vi "Test Stop.vi"(11 "Error in":errorcluster) -> (15 "Error out":errorcluster)   [LabVIEW 2020, in "CelsiusToFarenheitTests.lvlib"]
doc: "This VI is to validate the stop button"
uses:
  CelsiusToFarenheitTests.lvlib
  <vilib>/addons/_JKI Toolkits/Caraya/classes/Test Suite/Define Test Suite (JUnit Report).vi
  <vilib>/SLL Drona/APIs/Assert/AssertVI/AssertVIExecRunning.vi
  <vilib>/SLL Drona/APIs/Stimulus/ControlValue/SetValueAuto.vi
  <vilib>/SLL Drona/APIs/Assert/AssertVI/AssertVIExecIdle.vi
  <vilib>/SLL Drona/APIs/Stimulus/VI/CloseVI.vi
  <vilib>/addons/_JKI Toolkits/Caraya/classes/Test Suite/Test Suite.lvclass
  <vilib>/SLL Drona/Drona.lvlib
  <vilib>/addons/_JKI Toolkits/Caraya/classes/Test/Test.lvclass
  <vilib>/SLL Drona/APIs/Assert/AssertVI/AssertVI.lvlib
  <vilib>/SLL Drona/APIs/Stimulus/ControlValue/ControlValue.lvlib
  <vilib>/SLL Drona/APIs/Stimulus/VI/VI.lvlib
  <vilib>/Wiresmith Technology/G CLI/CLI Class/CLI.lvclass
panel:
  # "STOP BUTTON TEST"
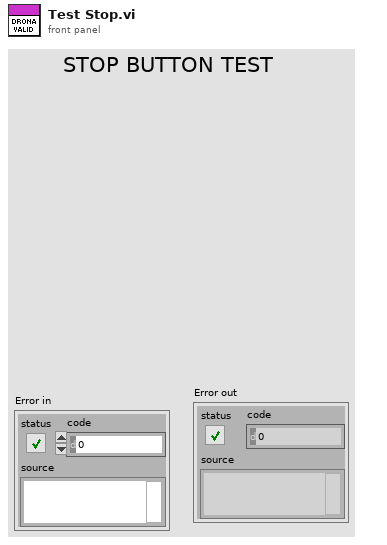
[diagram p1: front panel]
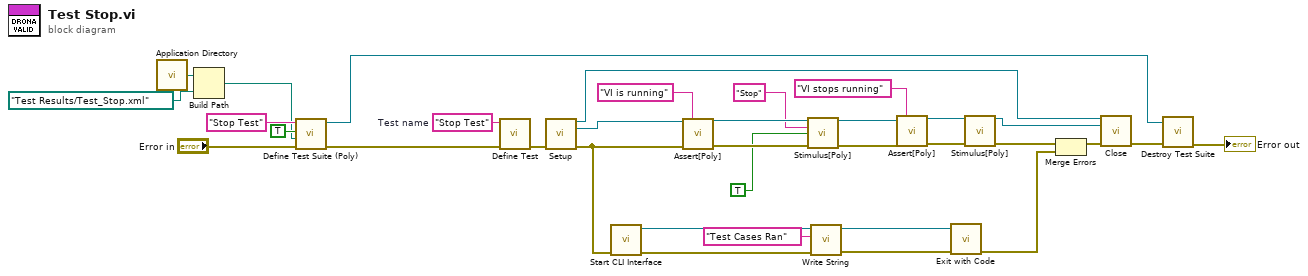
[diagram p0: block diagram]
diagram:
  w33 = "Stop Test"  # Test name
  n1 = call <vilib>:"Application Directory.vi"() -> ("Application Directory"=w3:path)
  n2 = Build Path(base path=w3, name or relative path=path "Test Results/Test_Stop.xml") -> (appended path=w1:path)
  n3 = call-poly <vilib>:"Define Test Suite (Poly).vi"("error in (no error)"="Error in", "Report Path"=w1, "Interactive"=TRUE, "Label (VI Title)"="Stop Test") -> ("error out"=w7:errorcluster, "Test Suite"=w4:refnum<class "Test Suite.lvclass">)  [unwired: 6 in]
  n4 = call <vilib>:"Define Test.vi"("error in (no error)"=w7, "Label (VI Title)"=w33) -> ("error out"=w34:errorcluster)  [unwired: 9 in]
  n5 = call <vilib>:"Setup.vi"("error in"=w34) -> ("Application Ref"=w32:refnum<vi>, "VI Reference Out"=w29:refnum<vi>, "error out"=w19:errorcluster)  [unwired: 12 in]
  n6 = call <vilib>:"Start CLI Interface.vi"("error in (no error)"=w19) -> ("error out"=w18:errorcluster, "CLI out"=w17:refnum<class "CLI.lvclass">)  [unwired: 7 in, 2 out]
  n7 = call-poly <vilib>:"Assert[Poly].vi"("VI Reference In"=w29, "Test Label"="VI is running", "Error In"=w19) -> ("VI Reference Out"=w27:refnum<vi>, "Error Out"=w28:errorcluster)  [unwired: 11 in]
  n8 = call-poly <vilib>:"Stimulus[Poly].vi"("VI Reference In"=w27, "Control Path"="Stop", "Value (Signaling)"=TRUE, "error in"=w28) -> ("VI Reference Out"=w23:refnum<vi>, "error out"=w24:errorcluster)  [unwired: 10 in]
  n9 = call <vilib>:"Write String.vi"("error in (no error)"=w18, "Text to Write"="Test Cases Ran", "CLI in"=w17) -> ("error out"=w14:errorcluster, "CLI out"=w15:refnum<class "CLI.lvclass">)  [unwired: 7 in]
  n10 = call-poly <vilib>:"Assert[Poly].vi"("VI Reference In"=w23, "Test Label"="VI stops running", "Error In"=w24) -> ("VI Reference Out"=w20:refnum<vi>, "Error Out"=w21:errorcluster)  [unwired: 11 in]
  n11 = call <vilib>:"Exit with Code.vi"("error in (no error)"=w14, "CLI in"=w15) -> ("error out"=w12:errorcluster)  [unwired: 9 in]
  n12 = call-poly <vilib>:"Stimulus[Poly].vi"("VI Reference In"=w20, "error in"=w21) -> ("VI Reference Out"=w31:refnum<vi>, "error out"=w13:errorcluster)  [unwired: 12 in]
  n13 = Merge Errors(w13, w12) -> (w11:errorcluster)
  n14 = call <vilib>:"Close.vi"("Application Ref"=w32, "VI Reference"=w31, "error in"=w11) -> ("error out"=w6:errorcluster)  [unwired: 12 in]
  n15 = call-dynamic "Destroy Test Suite.vi"("error in (no error)"=w6, "Test Suite in"=w4) -> ("error out"=→"Error out":errorcluster)  [unwired: 8 in, 1 out]
